vi "Test Helper Loop Broadcast Stopping Twice Times Out.vi"(8 "error in (no error)":errorcluster, 11 "Helper Loop Test In":refnum<class "Helper Loop Test.lvclass">) -> (0 "error out":errorcluster, 3 "Helper Loop Test Out":refnum<class "Helper Loop Test.lvclass">)   [LabVIEW 2020, in "Helper Loop Test.lvclass"]
uses:
  Helper Loop Test.lvclass
  C:/Program Files (x86)/National Instruments/LabVIEW 2020/vi.lib/Asteme/LUnit/Test Case.lvclass
  Mock Process/Mock Process.lvclass
  C:/Users/anton/Documents/GitHub/Triarc-Framework/source/Framework/Process/Process.lvclass
  <vilib>/Asteme/LUnit/Test Case.lvclass/Test Case.ctl
  <vilib>/Asteme/LUnit/LUnit Assertion Result.lvclass/LUnit Assertion Result.ctl
  Framework/Process/Process.lvclass/Process.ctl
  <vilib>/Asteme/LUnit/Set Assertion Type.vi
  <vilib>/Asteme/LUnit/Palette/Fail.vi
  <vilib>/Asteme/LUnit/Palette/Pass.vi
  Framework/Process/Public/Get Lifecycle State.vi
  Framework/Process/Private/SubVIs/Wait for finish.vi
  Framework/Process/Protected/Messaging/Enqueue Message.vi
  Framework/Process/Private/SubVIs/Set Lifecycle State.vi
  <vilib>/Asteme/LUnit/LUnit Write Assertion Type.vi
  <vilib>/Asteme/LUnit/Add test result.vi
  <vilib>/Asteme/LUnit/LUnit Write Passed.vi
  <vilib>/Asteme/LUnit/LUnit Get Test Case.vi
  <vilib>/Asteme/LUnit/LUnit Write Message.vi
  <vilib>/Asteme/LUnit/LUnit Write Description.vi
  <vilib>/Utility/error.llb/Clear Errors.vi
  <vilib>/Asteme/LUnit/Read Test Case Name.vi
  <vilib>/Asteme/LUnit/Assertion Result/LUnit Get Test Name.vi
  <vilib>/Utility/error.llb/Error Cluster From Error Code.vi
  <vilib>/Asteme/LUnit/LUnit Assertion Result.lvclass
  Framework/Process/Process.lvclass
  <vilib>/Asteme/LUnit/Test Case.lvclass
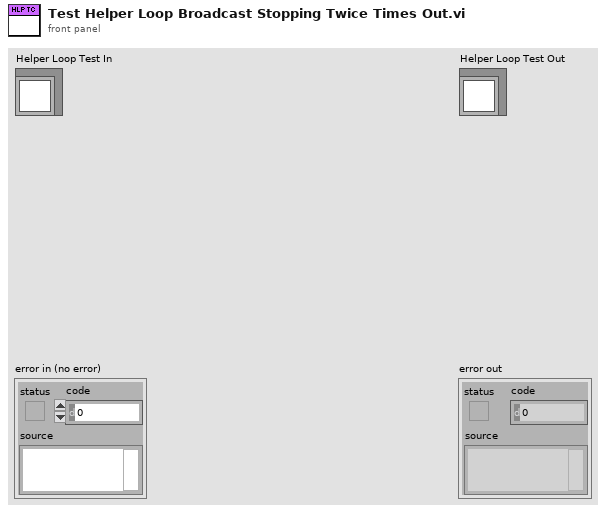
[diagram p1: front panel]
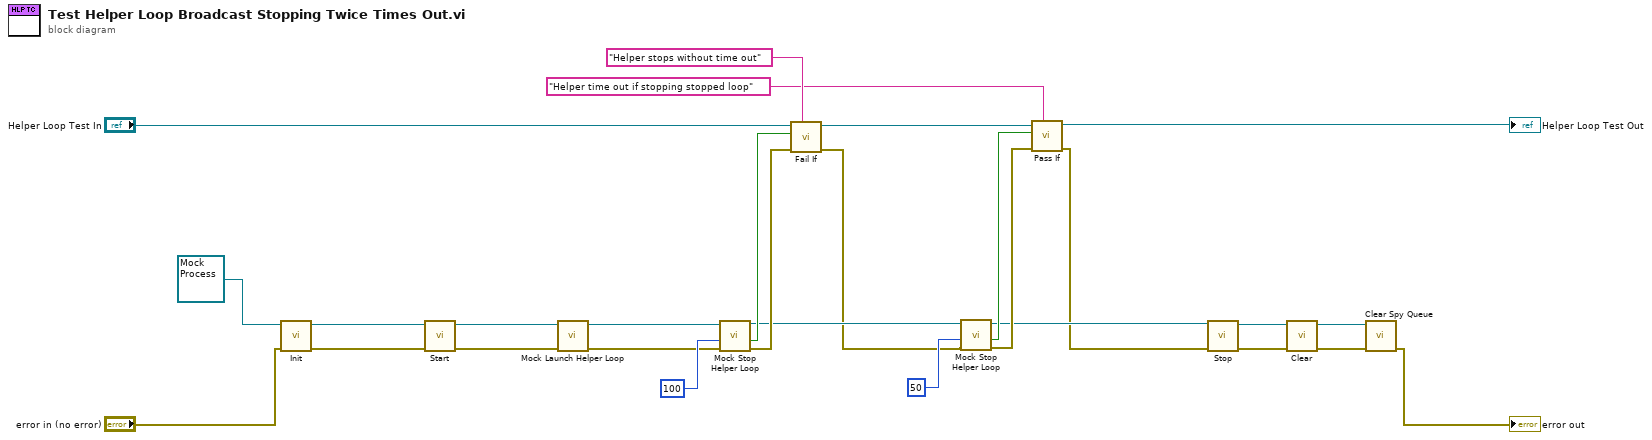
[diagram p0: block diagram]
diagram:
  n1 = call-dynamic "Init.vi"("error in (no error)"="error in (no error)", "Mock Process In"=refnum<class "Mock Process.lvclass"> refnum) -> ("error out"=w27:errorcluster, "Mock Process Out"=w28:refnum<class "Mock Process.lvclass">)  [unwired: 8 in]
  n2 = call "Start.vi"("error in (no error)"=w27, "Process In"=w28) -> ("error out"=w25:errorcluster, "Process Out"=w26:refnum<class "Mock Process.lvclass">)  [unwired: 8 in]
  n3 = call "Mock Launch Helper Loop.vi"("error in (no error)"=w25, "Mock Process in"=w26) -> ("error out"=w11:errorcluster, "Mock Process out"=w12:refnum<class "Mock Process.lvclass">)  [unwired: 8 in]
  n4 = call "Mock Stop Helper Loop.vi"("error in (no error)"=w11, "timeout in ms (-1)"=100, "Mock Process in"=w12) -> ("error out"=w24:errorcluster, "timed out?"=w13:bool, "Mock Process out"=w6:refnum<class "Mock Process.lvclass">)  [unwired: 6 in]
  n5 = call <vilib>:"Fail If.vi"("Description"="Helper stops without time out", "error in (no error)"=w24, "Fail?"=w13, "Test Case In"="Helper Loop Test In") -> ("error out"=w5:errorcluster, "Test Case Out"=w2:refnum<class "Helper Loop Test.lvclass">)  [unwired: 6 in]
  n6 = call "Mock Stop Helper Loop.vi"("error in (no error)"=w5, "timeout in ms (-1)"=50, "Mock Process in"=w6) -> ("error out"=w7:errorcluster, "timed out?"=w10:bool, "Mock Process out"=w4:refnum<class "Mock Process.lvclass">)  [unwired: 6 in]
  n7 = call <vilib>:"Pass If.vi"("Description"="Helper time out if stopping stopped loop", "error in (no error)"=w7, "Pass?"=w10, "Test Case In"=w2) -> ("error out"=w3:errorcluster, "Test Case Out"=→"Helper Loop Test Out":refnum<class "Helper Loop Test.lvclass">)  [unwired: 6 in]
  n8 = call "Stop.vi"("error in (no error)"=w3, "Process In"=w4) -> ("error out"=w22:errorcluster, "Process Out"=w23:refnum<class "Mock Process.lvclass">)  [unwired: 7 in, 1 out]
  n9 = call-dynamic "Clear.vi"("error in (no error)"=w22, "Mock Process In"=w23) -> ("error out"=w20:errorcluster, "Mock Process Out"=w21:refnum<class "Mock Process.lvclass">)  [unwired: 8 in]
  n10 = call-dynamic "Clear Spy Queue.vi"("error in (no error)"=w20, "Mock Process In"=w21) -> ("error out"=→"error out":errorcluster)  [unwired: 8 in, 1 out]
